vi "Configure Channel.vi"(0 "device session in":refnum<class "Device Session.lvclass">, 1 "enable channel (T)":bool=TRUE, 2 "range adjust":dbl=1.0 format="%#_6p", 5 "channels":u32[](array[numeric]), 7 "vertical range (Vpp)":dbl=1.0 format="%#_6p", 9 "vertical offset (V)":dbl format="%#_6p", 11 "error in":errorcluster, 12 "bandwidth":T1(ring), 13 "coupling":enum8{"Default", "DC", "AC"}(ring), 14 "impedance":enum8{"Default", "1 mega ohm", "50 ohm"}(ring)) -> (4 "device session out":refnum<class "Device Session.lvclass">, 15 "error out":errorcluster)   [LabVIEW 2021, in "Device Session.lvclass"]
doc: "Configures a channel with the specified parameters and uses the coerced configuration to compute and return the coefficients for a scaled fetch.\n\n<B>Input Parameters</B>\n\n<B>range adjust</B> adjusts the digital corrected data using the scaling factor. This can be used to prevent clipping when the acquired data is slightly greater than the nominal range.\n\n<B>enable channel (T)</B> enables or disables the channel. Setting this value to FALSE physically disconnects the channel.\n\n<B>device session in</B> is a reference to the Device Session object, which contains a session to each instrument design library used in this sample project. This parameter is obtained from the 'Open Session' VI.\n\n<B>channels</B> specifies the channels to be configured.\n\n<B>vertical range (Vpp)</B> specifies the peak-to-peak input range for the channel. The default value is 1 V.\n\n<B>vertical offset (V)</B> specifies in volts the location of the center of the 'vertical range' input with respect to ground.\n\n<B>bandwidth</B> specifies the bandwidth configuration for the channel.\n\n'Default': The default bandwidth setting for the device.\n'Full Bandwidth': No attenuation of the signal.\n'Anti-alias Filter': Attenuates unwanted high-frequency components of an analog signal prior to its conversion into a digital value. These signals would otherwise appear as undesired, aliased frequency components.\n\n<B>coupling</B> specifies the coupling configuration for the channel.\n\n'Default': The default coupling setting of the device.\n'DC': Direct Current signal components will not be attenuated.\n'AC': Alternating Current signal components will not be attenuated.\n\n<B>impedance</B> specifies the impedance configuration for the channel.\n\n'Default': The default impedance setting for the device.\n'1 MOhm': The impedance of the channel will be configured at 1 MOhm.\n'50 Ohm': The impedance of the channel will be configured at 50 Ohms.\n\n<B>error in</B> describes error conditions that occur before this node runs. This input provides standard 'error in' functionality.\n\n<B>Output Parameters</B>\n\n<B>device session out</B> passes a reference to the session to the next VI.\n\n<B>error out</B> contains error information. This output provides standard 'error out' functionality."
uses:
  Device Session.lvclass
  Device Session.lvclass/Device Session.ctl
  <instrlib>/HSAI-RIO/Types/v1/Host/Typedefs/Additional Channel Configuration.ctl
  <instrlib>/HSAI-RIO/Types/v1/Host/Typedefs/Bandwidth.ctl
  <instrlib>/HSAI-RIO/Types/v1/Host/Typedefs/Coupling.ctl
  <instrlib>/HSAI-RIO/Types/v1/Host/Typedefs/Impedance.ctl
  <instrlib>/HSAI-RIO/Config/Group A/v1/Host/Main/niHSAI Group A Config v1 Host.lvclass
  <instrlib>/HSAI-RIO/Types/v1/Host/niHSAI Types v1 Host.lvlib
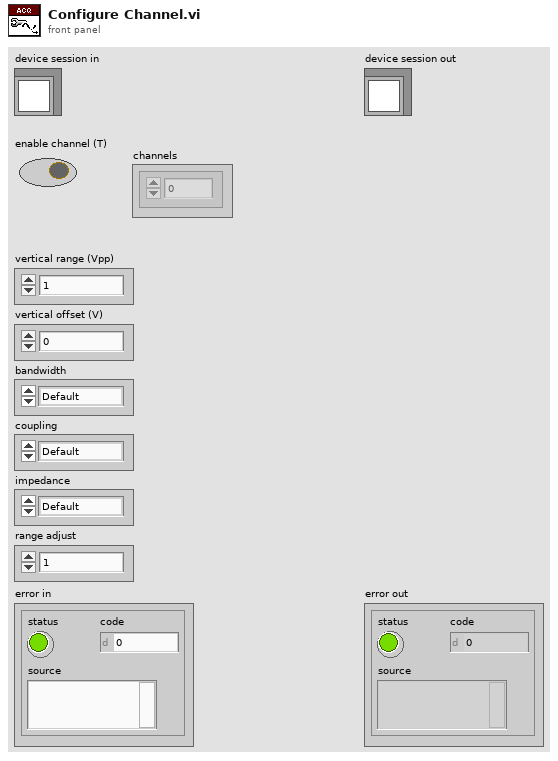
[diagram p1: front panel]
types:
  T1 = enum8{"Default", "Full Bandwidth", "Anti-alias Filter", "80 MHz FIR Filter", "40 MHz FIR Filter", "20 MHz FIR Filter"}
  T2 = typedef "niHSAI Types v1 Host.lvlib/Additional Channel Configuration.ctl" = cluster{"Bandwidth":T3, "Coupling":T4, "Impedance":T5}
  T3 = typedef "niHSAI Types v1 Host.lvlib/Bandwidth.ctl" = enum8{"Default", "Full Bandwidth", "Anti-alias Filter", "150 MHz"}
  T4 = typedef "niHSAI Types v1 Host.lvlib/Coupling.ctl" = enum8{"Default", "DC", "AC"}
  T5 = typedef "niHSAI Types v1 Host.lvlib/Impedance.ctl" = enum8{"Default", "1 mega ohm", "50 ohm"}
  T6 = typedef "Device Session.lvclass/Device Session Object.ctl" = cluster{"fpga reference":T7, "reg bus":refnum<class "niInstr FIFO Register Bus v1 Host.lvclass">, "subsystem map":refnum<class "niInstr Subsystem Map v1 Host.lvclass">, "cal data":refnum<class "niHSAI Cal Data v1 Host.lvclass">, "config":refnum<class "niHSAI Group A Config v1 Host.lvclass">, "acquisition 0":refnum<class "niInstr Multirecord Acquisition v1 Host.lvclass">, "acquisition 1":refnum<class "niInstr Multirecord Acquisition v1 Host.lvclass">, "number of selected acq channels":u8, "selected acq channels":bool[], "number of channels":u32, "configured channels":bool[], "acq configuration":cluster{"number of samples":u64, "number of records":u64, "pretrigger samples":u64}, "actual channel configuration":T8[], "sample clock rate (Hz)":dbl, "scaling coefficients":T9[]}
  T7 = typedef "Device Session.lvclass/FPGA Refnum.ctl" = refnum<k20>
  T8 = typedef "niHSAI Types v1 Host.lvlib/Channel Configuration.ctl" = cluster{"channel":u32, "coupling":T4, "impedance":T5, "bandwidth":T3, "vertical range":dbl, "vertical offset":dbl}
  T9 = typedef "niInstr Multirecord Acquisition v1 Host.lvclass/Scaling Coefficient.ctl" = cluster{"gain":dbl, "offset":dbl}
  T10 = typedef "niHSAI Types v1 Host.lvlib/Scaling Coefficients.ctl" = cluster{"gain":dbl, "offset":dbl}
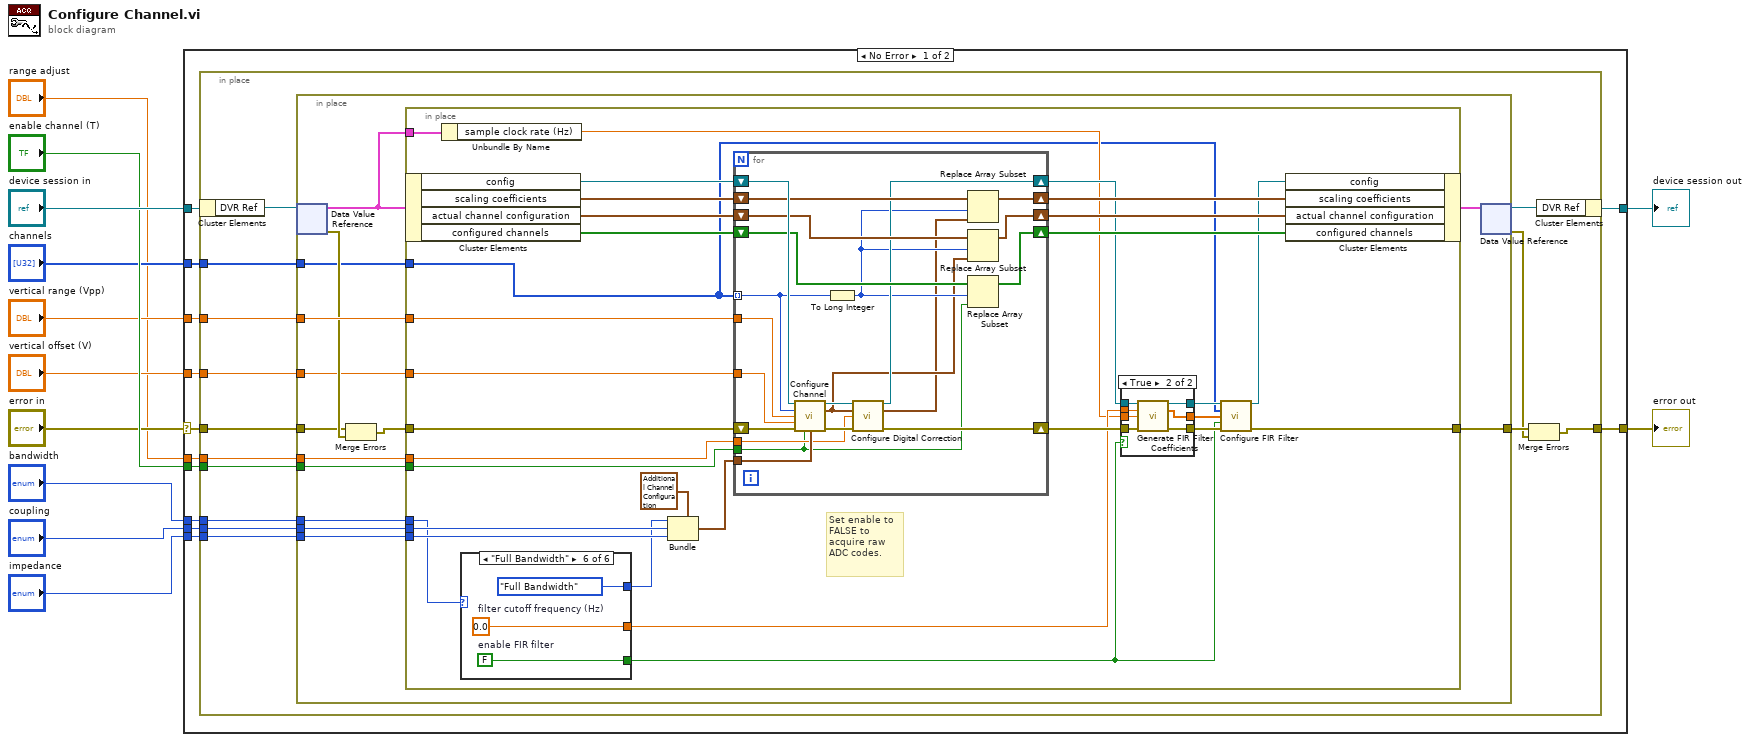
[diagram p0: block diagram]
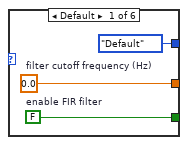
[diagram p2: hidden frame]
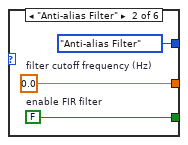
[diagram p3: hidden frame]
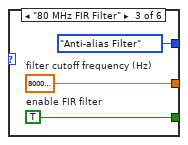
[diagram p4: hidden frame]
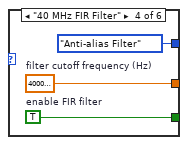
[diagram p5: hidden frame]
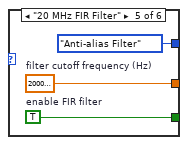
[diagram p6: hidden frame]
diagram:
  n1 = case shown="No Error" "error in" {
    selector: "error in" -> [w22 w132]
    tunnel: "device session in" -> [w14 w131]
    tunnel: [w13 w131] -> w11
    tunnel: "enable channel (T)" -> [w24 _]
    tunnel: "vertical range (Vpp)" -> [w23 _]
    tunnel: [w15 w132] -> w8
    tunnel: "channels" -> [w21 _]
    tunnel: "bandwidth" -> [w20 _]
    tunnel: "coupling" -> [w19 _]
    tunnel: "impedance" -> [w18 _]
    tunnel: "vertical offset (V)" -> [w17 _]
    tunnel: "range adjust" -> [w16 _]
    frame No Error {
      n2 = in-place {
        in-place-border: w24 -> [w38]
        in-place-border: w23 -> [w37]
        in-place-border: w22 -> [w36]
        in-place-border: w21 -> [w35]
        in-place-border: w20 -> [w32]
        in-place-border: w19 -> [w31]
        in-place-border: w18 -> [w30]
        in-place-border: w17 -> [w29]
        in-place-border: w16 -> [w28]
        in-place-border: [w27] -> w15
        n3 = in-place-cluster #1(w14) -> ("DVR Ref"=w26:refnum<data-value>)
        n4 = in-place {
          in-place-border: w38 -> [w48]
          in-place-border: w37 -> [w52]
          in-place-border: w36 -> [w50]
          in-place-border: [w49] -> w34
          in-place-border: w35 -> [w41]
          in-place-border: w32 -> [w45]
          in-place-border: w31 -> [w46]
          in-place-border: w30 -> [w47]
          in-place-border: w29 -> [w44]
          in-place-border: w28 -> [w43]
          n5 = in-place-dvr #2(w26) -> (w39:T6, w51:errorcluster)
          n6 = Merge Errors(w50, w51) -> (w42:errorcluster)
          n7 = in-place {
            in-place-border: w52 -> [w80]
            in-place-border: [w55] -> w49
            in-place-border: w48 -> [w71]
            in-place-border: w47 -> [w65]
            in-place-border: w46 -> [w66]
            in-place-border: w45 -> [w64]
            in-place-border: w44 -> [w82]
            in-place-border: w43 -> [w72]
            in-place-border: w42 -> [w81]
            in-place-border: w41 -> [w53]
            in-place-border: w39 -> [w61]
            # "Set enable to FALSE to acquire raw ADC codes."
            n8 = in-place-cluster #3(w39) -> ("config"=w79:refnum<class "niHSAI Group A Config v1 Host.lvclass">, "scaling coefficients"=w78:T9[], "actual channel configuration"=w76:T8[], "configured channels"=w75:bool[])
            n9 = Unbundle By Name(w61) -> ("sample clock rate (Hz)"=w60:dbl)
            n10 = case shown="\"Full Bandwidth\"" w64 {
              tunnel: [Bandwidth."Default" ("Bandwidth") Bandwidth."Anti-alias Filter" ("Bandwidth") Bandwidth."Anti-alias Filter" ("Bandwidth") Bandwidth."Anti-alias Filter" ("Bandwidth") Bandwidth."Anti-alias Filter" ("Bandwidth") Bandwidth."Full Bandwidth" ("Bandwidth")] -> w63
              tunnel: [w84 w87 w90 w93 w96 w99] -> w62
              tunnel: [w83 w86 w89 w92 w95 w98] -> w54
              frame Default {
                w83 = FALSE  # enable FIR filter
                w84 = 0.0  # filter cutoff frequency (Hz)
              }
              frame "Anti-alias Filter" {
                w86 = FALSE  # enable FIR filter
                w87 = 0.0  # filter cutoff frequency (Hz)
              }
              frame "80 MHz FIR Filter" {
                w89 = TRUE  # enable FIR filter
                w90 = 80000000.0  # filter cutoff frequency (Hz)
              }
              frame "40 MHz FIR Filter" {
                w92 = TRUE  # enable FIR filter
                w93 = 40000000.0  # filter cutoff frequency (Hz)
              }
              frame "20 MHz FIR Filter" {
                w95 = TRUE  # enable FIR filter
                w96 = 20000000.0  # filter cutoff frequency (Hz)
              }
              frame "Full Bandwidth" {
                w98 = FALSE  # enable FIR filter
                w99 = 0.0  # filter cutoff frequency (Hz)
              }
            }
            n11 = Bundle(cluster=T2 {"Bandwidth"=enum."Default", "Coupling"=enum."Default", "Impedance"=enum."Default"} ("additional channel configuration"), "Bandwidth"=w63, "Coupling"=w66, "Impedance"=w65) -> (w67:T2)
            n12 = for {
              tunnel: w82 -> [w127]
              tunnel: w80 -> [w125]
              tunnel: w53 -> [w122] mode=indexing
              tunnel: w67 -> [w115]
              tunnel: w72 -> [w114]
              tunnel: w71 -> [w111]
              shift-right: [w128] -> w70
              shift-left: w81 -> [w126]
              shift-right: [w116] -> w69
              shift-left: w79 -> [w124]
              shift-right: [w121] -> w77
              shift-left: w78 -> [w123]
              shift-right: [w117] -> w73
              shift-left: w76 -> [w120]
              shift-right: [w118] -> w74
              shift-left: w75 -> [w119]
              n13 = call-dynamic "Configure Channel.vi"("session in"=w124, "channel"=w122, "vertical range (V)"=w125, "vertical offset (V)"=w127, "error in"=w126, "enable channel (T)"=w111, "additional channel configuration"=w115) -> ("session out"=w130:refnum<class "niHSAI Group A Config v1 Host.lvclass">, "actual channel configuration"=w112:T8, "error out"=w129:errorcluster)  [unwired: 5 in, 1 out]
              n14 = To Long Integer(number=w122) -> (32bit integer=w113:i32)
              n15 = call-dynamic "Configure Digital Correction.vi"("session in"=w130, "actual channel configuration"=w112, "range adjust"=w114, "error in"=w129) -> ("session out"=w116:refnum<class "niHSAI Group A Config v1 Host.lvclass">, "scaling coefficients"=w110:T10, "error out"=w128:errorcluster)  [unwired: 9 in]
              n16 = Replace Array Subset(array=w123, new element=w110, index=w113) -> (w121:T9[])
              n17 = Replace Array Subset(array=w120, new element=w112, index=w113) -> (w117:T8[])
              n18 = Replace Array Subset(array=w119, new element=w111, index=w113) -> (w118:bool[])
            }
            n19 = case shown="True" w54 {
              tunnel: w70 -> [w102 w109]
              tunnel: w69 -> [w101 w108]
              tunnel: w62 -> [_ w107]
              tunnel: [w102 w106] -> w59
              tunnel: [w101 w105] -> w58
              tunnel: w60 -> [_ w104]
              tunnel: [_ w103] -> w57
              frame False {
              }
              frame True {
                n20 = call-dynamic "Generate FIR Filter Coefficients.vi"("session in"=w108, "filter cutoff frequency (Hz)"=w107, "actual adc clock rate (Hz)"=w104, "error in"=w109) -> ("session out"=w105:refnum<class "niHSAI Group A Config v1 Host.lvclass">, "filter coefficients"=w103:dbl[], "error out"=w106:errorcluster)  [unwired: 9 in]
              }
            }
            n21 = call-dynamic "Configure FIR Filter.vi"("session in"=w58, "channels"=w53, "filter coefficients"=w57, "enable filter (T)"=w54, "error in"=w59) -> ("session out"=w56:refnum<class "niHSAI Group A Config v1 Host.lvclass">, "error out"=w55:errorcluster)  [unwired: 9 in]
            n22 = in-place-cluster #3("config"=w56, "scaling coefficients"=w77, "actual channel configuration"=w73, "configured channels"=w74) -> (w40:T6)
          }
          n23 = in-place-dvr #2(w40) -> (w25:refnum<data-value>, w33:errorcluster)
        }
        n24 = Merge Errors(w34, w33) -> (w27:errorcluster)
        n25 = in-place-cluster #1("DVR Ref"=w25) -> (w13:refnum<class "Device Session.lvclass">)
      }
    }
    frame Error {
    }
  }
  "error out" <- w8
  "device session out" <- w11
